vi "VerifyTriggerSource.vi"(8 "error in (no error)":errorcluster, 11 "TriggerSource":string) -> (0 "error out":errorcluster, 3 "DAQmx Terminal":tag)   [LabVIEW 2014, in "FGenPlugins.lvlib" / "NiPxi6733.lvclass"]
uses:
  NiPxi6733.lvclass
  <vilib>/Utility/error.llb/Error Cluster From Error Code.vi
  <vilib>/ErrorRing/Error Ring.xnode
  <resource>/objmgr/daqmx.rc
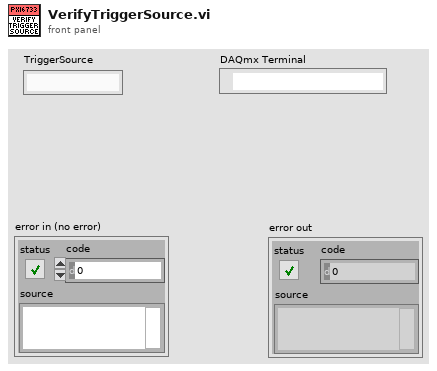
[diagram p1: front panel]
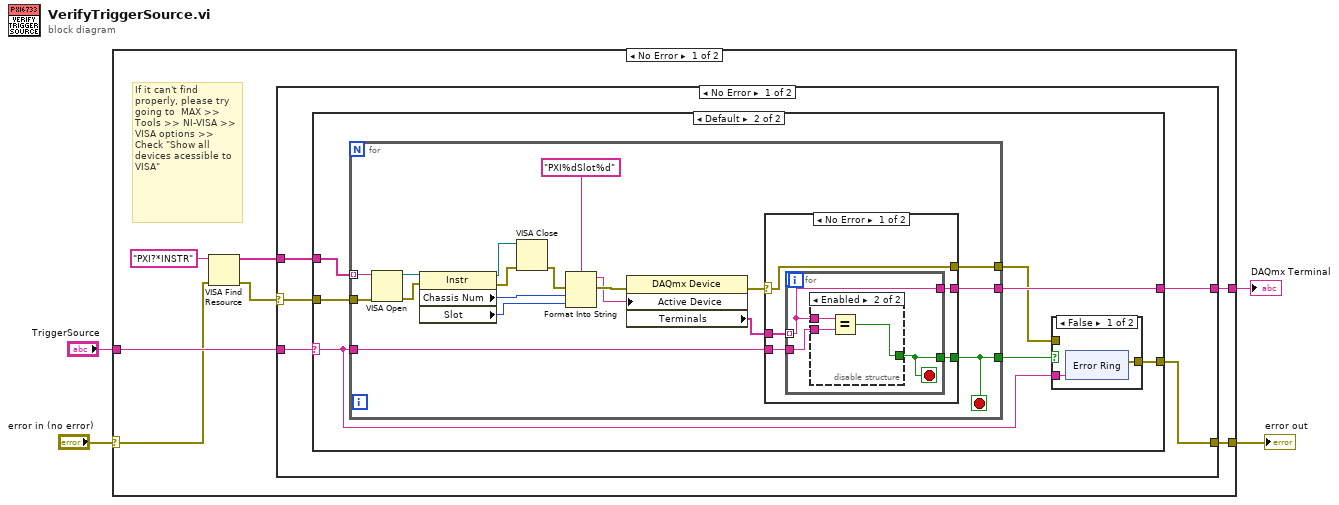
[diagram p0: block diagram]
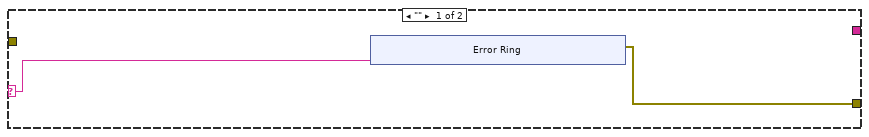
[diagram p2: hidden frame]
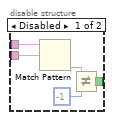
[diagram p4: hidden frame]
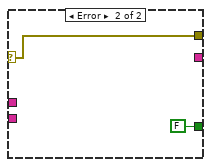
[diagram p5: hidden frame]
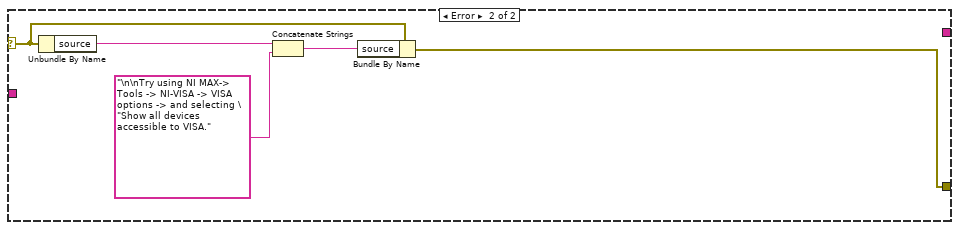
[diagram p6: hidden frame]
diagram:
  n1 = case shown="No Error" "error in (no error)" {
    selector: "error in (no error)" -> [w5 w84]
    tunnel: [w10 w84] -> w4
    tunnel: "TriggerSource" -> [w9 _]
    tunnel: [w8 _] -> w1
    frame No Error {
      # "If it can't find properly, please try going to  MAX >> Tools >> NI-VISA >> VISA options >> Check \"Show all devices acessible to VISA\""
      n2 = VISA Find Resource(8:w5, 11:"PXI?*INSTR" ("expression (\"?*\")")) -> (0:w11:errorcluster, 3:w7:string[])  [unwired: 1 in, 1 out]
      n3 = case shown="No Error" w11 {
        selector: w11 -> [w16 w81]
        tunnel: [w12 w79] -> w10
        tunnel: w9 -> [w15 _]
        tunnel: [w14 _] -> w8
        tunnel: w7 -> [w13 _]
        frame No Error {
          n4 = case shown="Default" w15 {
            selector: w15 -> [w17 w30]
            tunnel: w16 -> [_ w32]
            tunnel: [_ w29] -> w14
            tunnel: w13 -> [_ w28]
            tunnel: [w18 w26] -> w12
            frame "" {
              n5 = xnode "Error Ring"("parameter 0"=w17) -> ("error out"=w18:errorcluster)
            }
            frame Default {
              n6 = for {
                tunnel: w30 -> [w53]
                tunnel: [w43] -> w27
                tunnel: w32 -> [w52]
                tunnel: [w51] -> w31
                tunnel: [w50] -> w29
                tunnel: w28 -> [w46] mode=indexing
                stop <- w51 stop-if-true
                n7 = VISA Open(error in (no error)=w52, VISA resource name=w46) -> (VISA resource name=w60:refnum<visa-resource-name>, error out=w59:errorcluster)  [unwired: 3 in]
                n8 = property class="Instr"(reference=w60, error in=w59) -> (reference out=w57:refnum<visa-resource-name>, error out=w56:errorcluster, "Chassis Num"=w58:i16, "Slot"=w47:i16)
                n9 = VISA Close(VISA resource name=w57, error in (no error)=w56) -> (error out=w55:errorcluster)
                n10 = Format Into String(format string="PXI%dSlot%d" ("initial string"), error in=w55, w58, w47) -> (resulting string=w45:string, error out=w48:errorcluster)  [unwired: 1 in]
                n11 = property class="DAQmx Device"(error in=w48, "Active Device"=w45) -> (error out=w44:errorcluster, "Terminals"=w54:tag[])  [unwired: 1 in, 1 out]
                n12 = case shown="No Error" w44 {
                  selector: w44 -> [w61 w77]
                  tunnel: w54 -> [w65 _]
                  tunnel: w53 -> [w64 _]
                  tunnel: [w63 FALSE] -> w51
                  tunnel: [w62 _] -> w50
                  tunnel: [w61 w77] -> w43
                  frame No Error {
                    n13 = for {
                      tunnel: w65 -> [w66] mode=indexing
                      tunnel: w64 -> [w68]
                      tunnel: [w67] -> w63
                      tunnel: [w66] -> w62
                      stop <- w67 stop-if-true
                      n14 = disable-structure shown="Enabled" {
                        disable-tunnel: w68 -> [w71 w76]
                        disable-tunnel: [w70 w74] -> w67
                        disable-tunnel: w66 -> [w69 w75]
                        frame Disabled {
                          n15 = Match Pattern(string=w69, regular expression=w71) -> (offset past match=w72:i32)  [unwired: 1 in, 3 out]
                          n16 = Not Equal?(x=w72, y=-1) -> (x != y?=w70:bool)
                        }
                        frame Enabled {
                          n17 = Equal?(x=w75, y=w76) -> (x = y?=w74:bool)
                        }
                      }
                    }
                  }
                  frame Error {
                  }
                }
              }
              n18 = case shown="False" w31 {
                tunnel: w30 -> [w34 _]
                tunnel: [w33 w42] -> w26
                tunnel: w27 -> [_ w42]
                frame False {
                  n19 = xnode "Error Ring"("parameter 0"=w34) -> ("error out"=w33:errorcluster)
                }
                frame True {
                }
              }
            }
          }
        }
        frame Error {
          n20 = Unbundle By Name(w81) -> ("source"=w83:string)
          n21 = Concatenate Strings(w83, "\n\nTry using NI MAX-> Tools -> NI-VISA -> VISA options -> and selecting \"Show all devices accessible to VISA." ("string")) -> (w80:string)
          n22 = Bundle By Name(cluster=w81, "source"=w80) -> (w79:errorcluster)
        }
      }
    }
    frame Error {
    }
  }
  "error out" <- w4
  "DAQmx Terminal" <- w1
